vi "Test Tree Handlr API.vi"() -> ()   [LabVIEW 2023]
doc: "Tree Handlr allows opt-open close of all items in tree, and has a method for restoring the open/close state of tree items. Thus, if a tree must be udpated, but you want the open items to be retained, so can call teh approprioate method."
uses:
  <vilib>/Utility/error.llb/DialogType.ctl
  Tree Handlr.lvlib
panel:
  in  "Record Open Items":bool
  out "New Module Ring Value":i32=-1
  in  "Close All":bool
  in  "Restore Open Items":bool
  in  "Main Tree":string[](tree)
  out "last error":errorcluster
  in  "Show Diagram on Init":bool
  in  "Run as Singleton?":bool
  in  "Show Block Diagram":bool
  in  "Refresh Modules":bool
  out "Active Modules":string[](array[string])
  in  "Stop Module":bool
  in  "Select Module":i32(ring)=-1 caption="Select Module\nTo send Request to" items=["All"=-1]
  in  "Run New Module":bool
  in  "Hide Module Panel":bool
  in  "Show Module Panel":bool
  out "Status":string
  # "This VI tests the API for the Module."
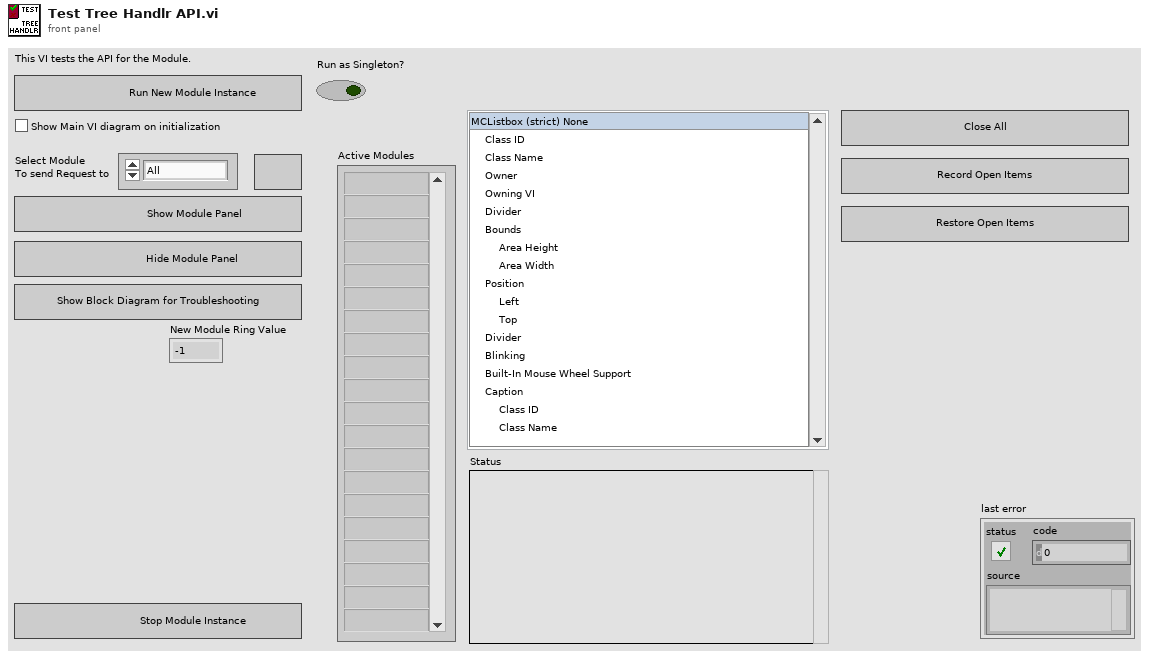
[diagram p1: front panel]
types:
  T1 = typedef "Tree Handlr.lvlib/Broadcast Events--cluster.ctl" = cluster{"Module Did Init":refnum<user-event>, "Status Updated":refnum<user-event>, "Error Reported":refnum<user-event>, "Module Did Stop":refnum<user-event>, "Update Module Execution Status":refnum<user-event>}
  T2 = typedef "DialogType.ctl" = u16
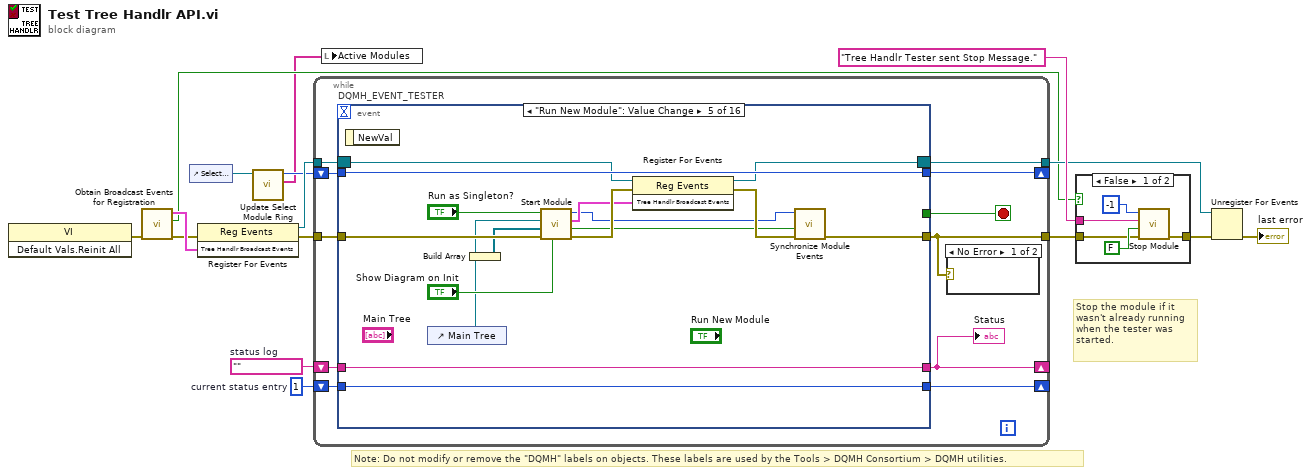
[diagram p0: block diagram]
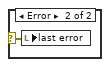
[diagram p3: hidden frame]
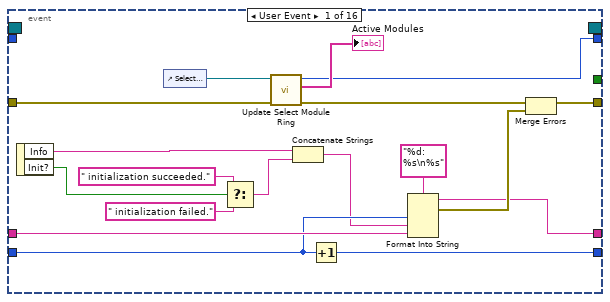
[diagram p4: hidden frame]
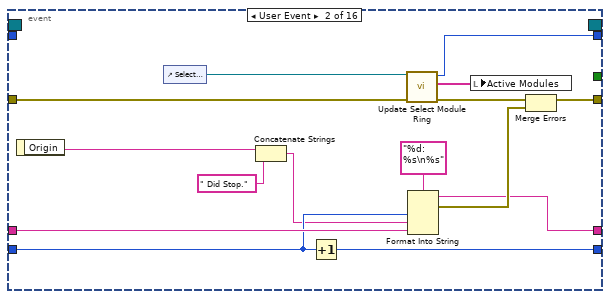
[diagram p5: hidden frame]
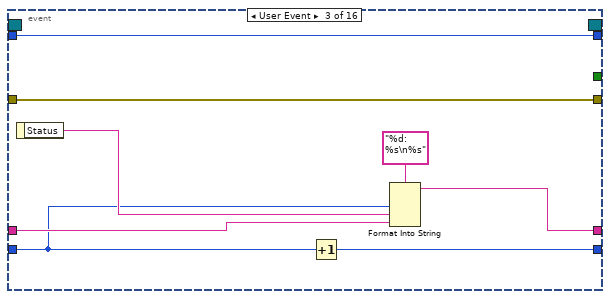
[diagram p6: hidden frame]
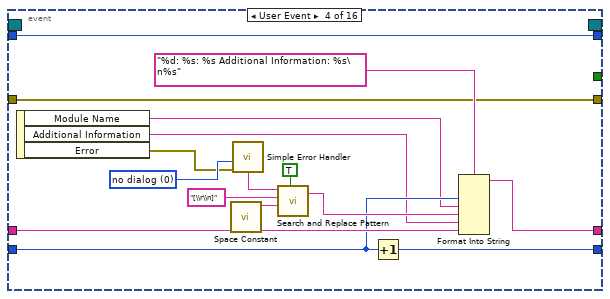
[diagram p7: hidden frame]
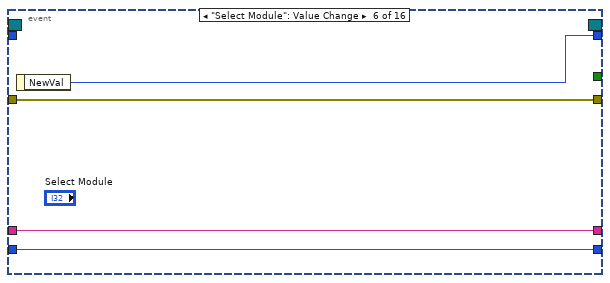
[diagram p8: hidden frame]
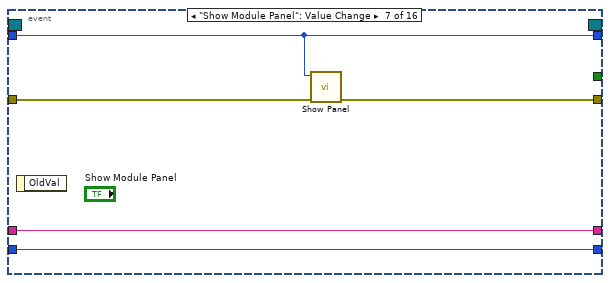
[diagram p9: hidden frame]
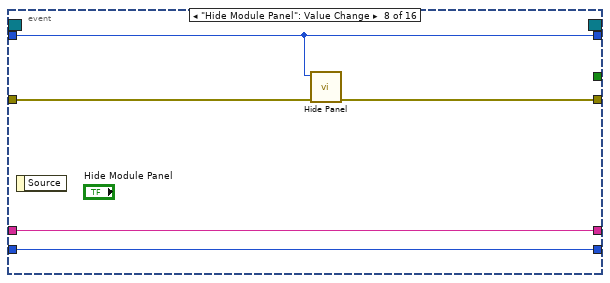
[diagram p10: hidden frame]
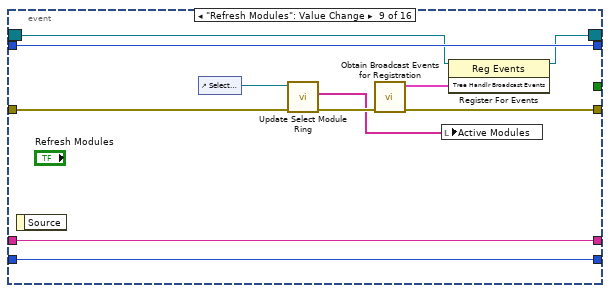
[diagram p11: hidden frame]
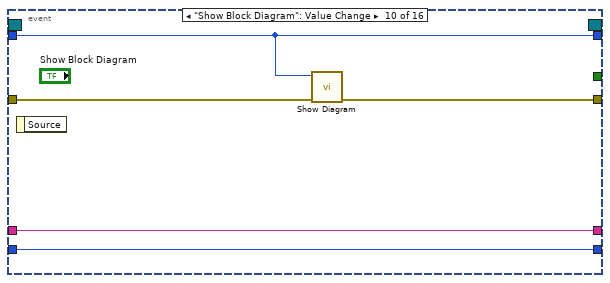
[diagram p12: hidden frame]
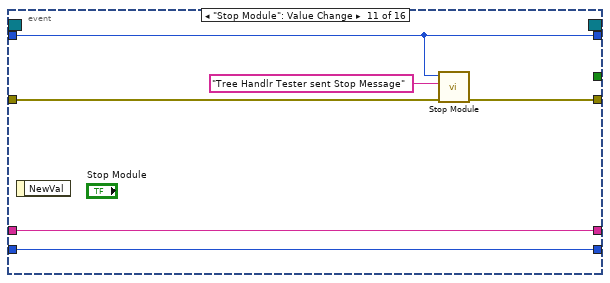
[diagram p13: hidden frame]
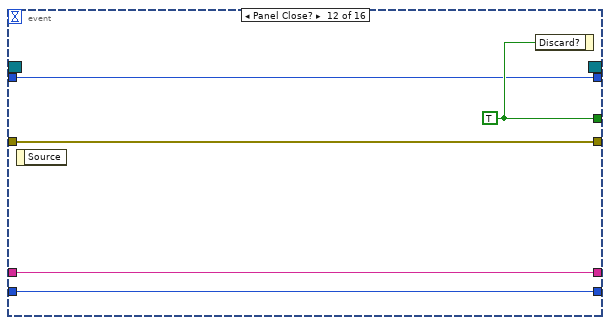
[diagram p14: hidden frame]
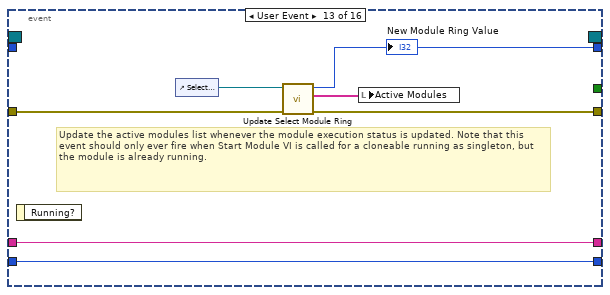
[diagram p15: hidden frame]
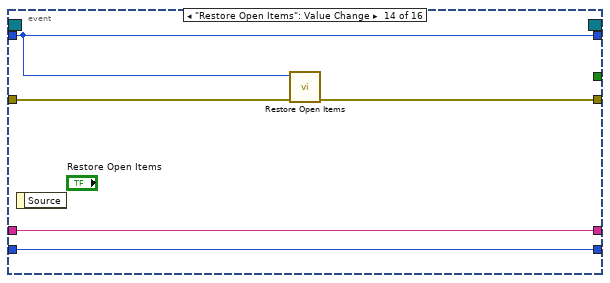
[diagram p16: hidden frame]
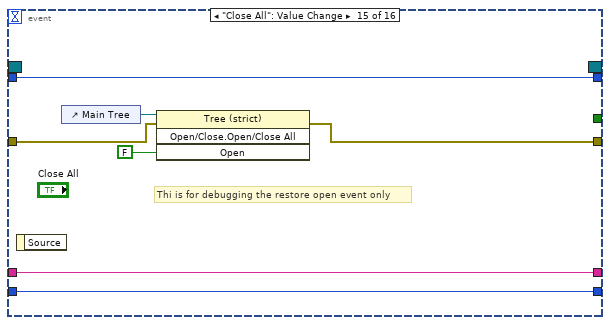
[diagram p17: hidden frame]
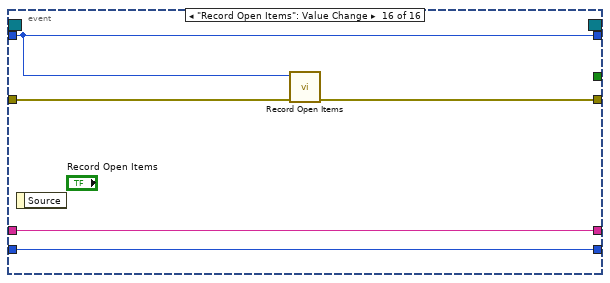
[diagram p18: hidden frame]
diagram:
  w13 = 1  # current status entry
  w14 = ""  # status log
  # "Stop the module if it wasn't already running when the tester was started."
  # "Note: Do not modify or remove the \"DQMH\" labels on objects. These labels are used by the Tools > DQMH Consortium > DQMH utilities."
  n1 = invoke class="VI" method="Default Vals.Reinit All"() -> (error out=w8:errorcluster)  [unwired: 3 in, 2 out]
  n2 = call "Obtain Broadcast Events for Registration.vi"("error in"=w8) -> ("error out"=w7:errorcluster, "Already running?"=w6:bool, "Tree Handlr Broadcast Events"=w12:T1)  [unwired: 8 in]
  n3 = control-ref of="Select Module"() -> (w3:refnum<vi>)
  n4 = register-events(error in=w7, w12) -> (reference out=w16:refnum<event-registration>, error out=w11:errorcluster)  [unwired: 1 in]
  n5 = call "Update Select Module Ring.vi"("Select Module Ring Ref"=w3) -> ("Active Modules (Array)"=w1:string[], "New Module Ring Value"=w2:i32)  [unwired: 8 in, 1 out]
  n6 = while {
    tunnel: w16 -> [w27]
    tunnel: [w18] -> w5
    tunnel: w11 -> [w26]
    shift-right: [w22] -> _
    shift-left: w14 -> [w24]
    shift-right: [w23] -> _
    shift-left: w13 -> [w25]
    shift-right: [w20] -> _
    shift-left: w2 -> [w21]
    tunnel: [w19] -> w9
    stop <- w17 stop-if-true
    n7 = event "DQMH_EVENT_TESTER" shown="[4] \"Run New Module\": Value Change" {
      selector: w27 -> [_ _ _ _ w95 _ _ _ w121 _ _ _ _ _ _ _]
      dyn-events: [_ _ _ _ w94 _ _ _ w120 _ _ _ _ _ _ _] -> w19
      timeout: _ -> [_ _ _ _ _ _ _ _ _ _ _ _ _ _ _ _]
      tunnel: [_ _ _ _ _ _ _ _ _ _ _ w142 _ _ _ _] -> w17
      tunnel: [w36 w53 w69 w73 w93 w105 w109 w114 w117 w128 w133 w138 w145 w150 w156 w162] -> w18
      tunnel: w26 -> [w38 w55 w69 w73 w96 w105 w110 w115 w122 w131 w134 w138 w146 w154 w155 w166]
      tunnel: w25 -> [w43 w58 w62 w76 w98 w103 w107 w112 w125 w129 w136 w140 w148 w152 w160 w164]
      tunnel: w24 -> [w44 w59 w65 w77 w99 w104 w108 w113 w126 w130 w137 w141 w149 w153 w161 w165]
      tunnel: [w41 w56 w66 w75 w99 w104 w108 w113 w126 w130 w137 w141 w149 w153 w161 w165] -> w22
      tunnel: [w42 w57 w68 w74 w98 w103 w107 w112 w125 w129 w136 w140 w148 w152 w160 w164] -> w23
      tunnel: w21 -> [_ _ w63 w85 w97 _ w106 w111 w124 w127 w135 w139 _ w151 w159 w163]
      tunnel: [w33 w50 w63 w85 w97 w102 w106 w111 w124 w127 w135 w139 w143 w151 w159 w163] -> w20
      event User Event {
        n8 = event-data() -> ("Info"=w40:string, "Init?"=w30:bool)  [unwired: 1 in]
        n9 = control-ref of="Select Module"() -> (w35:refnum<vi>)
        n10 = Select(t=" initialization succeeded.", s=w30, f=" initialization failed.") -> (s? t:f=w29:string)
        n11 = call "Update Select Module Ring.vi"("error in"=w38, "Select Module Ring Ref"=w35) -> ("error out"=w37:errorcluster, "Active Modules (Array)"=→"Active Modules":string[], "New Module Ring Value"=w33:i32)  [unwired: 7 in]
        n12 = Concatenate Strings(w40, w29) -> (w39:string)
        n13 = Increment(x=w43) -> (x+1=w42:i32)
        n14 = Format Into String(format string="%d: %s\n%s", w43, w39, w44) -> (resulting string=w41:string, error out=w46:errorcluster)  [unwired: 2 in]
        n15 = Merge Errors(w37, w46) -> (w36:errorcluster)
      }
      event User Event {
        n16 = event-data() -> ("Origin"=w48:string)  [unwired: 1 in]
        n17 = control-ref of="Select Module"() -> (w52:refnum<vi>)
        n18 = Concatenate Strings(w48, " Did Stop.") -> (w47:string)
        n19 = Increment(x=w58) -> (x+1=w57:i32)
        n20 = call "Update Select Module Ring.vi"("error in"=w55, "Select Module Ring Ref"=w52) -> ("error out"=w54:errorcluster, "Active Modules (Array)"=w51:string[], "New Module Ring Value"=w50:i32)  [unwired: 7 in]
        n21 = Format Into String(format string="%d: %s\n%s", w58, w47, w59) -> (resulting string=w56:string, error out=w61:errorcluster)  [unwired: 2 in]
        n22 = local write "Active Modules"(w51) -> ()
        n23 = Merge Errors(w54, w61) -> (w53:errorcluster)
      }
      event User Event {
        n24 = event-data() -> ("Status"=w64:string)  [unwired: 1 in]
        n25 = Increment(x=w62) -> (x+1=w68:i32)
        n26 = Format Into String(format string="%d: %s\n%s", w62, w64, w65) -> (resulting string=w66:string)  [unwired: 2 in, 1 out]
      }
      event User Event {
        w78 = T2 0 items=["no dialog", "OK message", "continue or stop message", "OK message + warnings", "continue/stop + warnings"] ("type of dialog (OK msg:1)")
        n27 = event-data() -> ("Module Name"=w72:string, "Additional Information"=w71:string, "Error"=w70:errorcluster)  [unwired: 1 in]
        n28 = call <vilib>:"Space Constant.vi"() -> ("String"=w82:string)
        n29 = call <vilib>:"Simple Error Handler.vi"("type of dialog (OK msg:1)"=w78, "error in (no error)"=w70) -> ("message"=w79:string)  [unwired: 3 in, 4 out]
        n30 = call <vilib>:"Search and Replace Pattern.vi"("string"=w79, "regular expression (\"\")"="[\\r\\n]" ("regular expression (\"\")"), "replace string (\"\")"=w82, "replace all? (F)"=TRUE ("replace all CR/LF with spaces")) -> ("result string"=w80:string)  [unwired: 1 in, 1 out]
        n31 = Increment(x=w76) -> (x+1=w74:i32)
        n32 = Format Into String(format string="%d: %s: %s Additional Information: %s\n%s", w76, w72, w80, w71, w77) -> (resulting string=w75:string)  [unwired: 2 in, 1 out]
      }
      event "Run New Module": Value Change {
        n33 = event-data() -> ()  [unwired: 1 in, 1 out]
        n34 = control-ref of="Main Tree"() -> (w87:refnum<vi>)
        n35 = Build Array(w87) -> (w86:refnum<vi>[])
        n36 = call "Start Module.vi"("Show Main VI Diagram on Init (F)"="Show Diagram on Init", "error in"=w96, "Tree Sync Refs"=w86, "Tree Ref"=w87, "Run as Singleton? (F)"="Run as Singleton?") -> ("error out"=w100:errorcluster, "Wait for Event Sync?"=w92:bool, "Tree Handlr Broadcast Events"=w91:T1, "Module ID"=w88:i32)  [unwired: 3 in]
        n37 = register-events(reference=w95, error in=w100, w91) -> (reference out=w94:refnum<event-registration>, error out=w101:errorcluster)
        n38 = call "Synchronize Module Events.vi"("error in"=w101, "Wait for Event Sync?"=w92, "Module ID in"=w88) -> ("error out"=w93:errorcluster)  [unwired: 7 in, 1 out]
      }
      event "Select Module": Value Change {
        n39 = event-data() -> ("NewVal"=w102:i32)  [unwired: 1 in]
      }
      event "Show Module Panel": Value Change {
        n40 = event-data() -> ()  [unwired: 1 in, 1 out]
        n41 = call "Show Panel.vi"("error in"=w110, "Module ID"=w106) -> ("error out"=w109:errorcluster)  [unwired: 9 in]
      }
      event "Hide Module Panel": Value Change {
        n42 = event-data() -> ()  [unwired: 1 in, 1 out]
        n43 = call "Hide Panel.vi"("error in"=w115, "Module ID"=w111) -> ("error out"=w114:errorcluster)  [unwired: 9 in]
      }
      event "Refresh Modules": Value Change {
        n44 = event-data() -> ()  [unwired: 1 in, 1 out]
        n45 = control-ref of="Select Module"() -> (w123:refnum<vi>)
        n46 = call "Update Select Module Ring.vi"("error in"=w122, "Select Module Ring Ref"=w123) -> ("error out"=w118:errorcluster, "Active Modules (Array)"=w116:string[])  [unwired: 7 in, 1 out]
        n47 = call "Obtain Broadcast Events for Registration.vi"("error in"=w118) -> ("error out"=w117:errorcluster, "Tree Handlr Broadcast Events"=w119:T1)  [unwired: 8 in, 1 out]
        n48 = local write "Active Modules"(w116) -> ()
        n49 = register-events(reference=w121, w119) -> (reference out=w120:refnum<event-registration>)  [unwired: 1 in, 1 out]
      }
      event "Show Block Diagram": Value Change {
        n50 = event-data() -> ()  [unwired: 1 in, 1 out]
        n51 = call "Show Diagram.vi"("error in"=w131, "Module ID"=w127) -> ("error out"=w128:errorcluster)  [unwired: 9 in]
      }
      event "Stop Module": Value Change {
        n52 = event-data() -> ()  [unwired: 1 in, 1 out]
        n53 = call "Stop Module.vi"("error in"=w134, "Origin"="Tree Handlr Tester sent Stop Message", "Module ID"=w135) -> ("error out"=w133:errorcluster)  [unwired: 8 in]
      }
      event Panel Close? {
        w142 = TRUE ("Discard?")
        n54 = event-data() -> ()  [unwired: 1 in, 1 out]
        n55 = event-data("Discard?"=w142) -> ()  [unwired: 1 in, 1 out]
      }
      event User Event {
        # "Update the active modules list whenever the module execution status is updated. Note that this event should only ever fire when Start Module VI is called for a cloneable running as singleton, but the module is already running."
        n56 = event-data() -> ()  [unwired: 1 in, 1 out]
        n57 = control-ref of="Select Module"() -> (w147:refnum<vi>)
        n58 = call "Update Select Module Ring.vi"("error in"=w146, "Select Module Ring Ref"=w147) -> ("error out"=w145:errorcluster, "Active Modules (Array)"=w144:string[], "New Module Ring Value"=w143:i32)  [unwired: 7 in]
        "New Module Ring Value" <- w143
        n59 = local write "Active Modules"(w144) -> ()
      }
      event "Restore Open Items": Value Change {
        n60 = event-data() -> ()  [unwired: 1 in, 1 out]
        n61 = call "Restore Open Items.vi"("error in"=w154, "Module ID"=w151) -> ("error out"=w150:errorcluster)  [unwired: 9 in]
      }
      event "Close All": Value Change {
        # "Thi is for debugging the restore open event only"
        n62 = event-data() -> ()  [unwired: 1 in, 1 out]
        n63 = control-ref of="Main Tree"() -> (w158:refnum<vi>)
        n64 = invoke class="Tree (strict)" method="Open/Close.Open/Close All"(reference=w158, error in=w155, "Open"=FALSE ("Open?")) -> (error out=w156:errorcluster)  [unwired: 1 in, 3 out]
      }
      event "Record Open Items": Value Change {
        n65 = event-data() -> ()  [unwired: 1 in, 1 out]
        n66 = call "Record Open Items.vi"("error in"=w166, "Module ID"=w163) -> ("error out"=w162:errorcluster)  [unwired: 9 in]
      }
    }
    "Status" <- w22
    n67 = case shown="No Error" w18 {
      selector: w18 -> [_ w28]
      frame No Error {
      }
      frame Error {
        n68 = local write "last error"(w28) -> ()
      }
    }
  }
  n69 = local write "Active Modules"(w1) -> ()
  n70 = case shown="False" w6 {
    tunnel: [w171 w172] -> w15
    tunnel: "Tree Handlr Tester sent Stop Message." ("Origin") -> [w170 _]
    tunnel: w5 -> [w167 w172]
    frame False {
      n71 = call "Stop Module.vi"("error in"=w167, "Wait for Module to stop? (F)"=FALSE ("Wait for Module to stop?"), "Origin"=w170, "Module ID"=-1 ("Stop all")) -> ("error out"=w171:errorcluster)  [unwired: 7 in]
    }
    frame True {
    }
  }
  n72 = Unregister For Events(event registration refnum=w9, error in=w15) -> (error out=→"last error":errorcluster)
